vi "WriteConsumerState.vi"(8 "error in (no error)":errorcluster, 10 "Consumer State":string, 11 "Queue in":refnum<queue>) -> (0 "error out":errorcluster, 3 "Queue out":refnum<queue>)   [LabVIEW 2019]
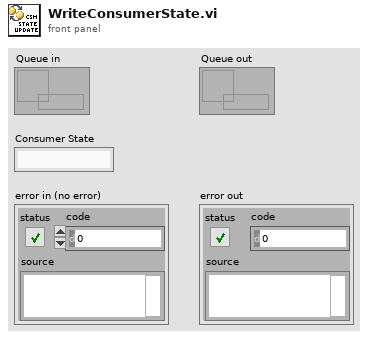
[diagram p1: front panel]
types:
  T1 = cluster{"Consumer State":string, "RxData":string, "error constant":errorcluster}
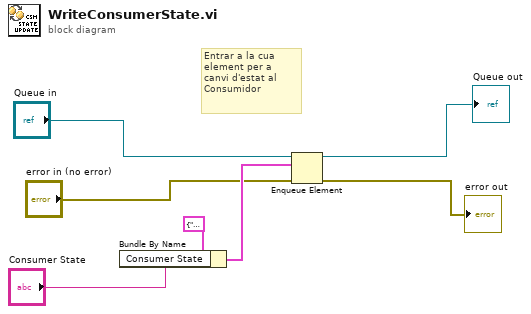
[diagram p0: block diagram]
diagram:
  # "Entrar a la cua element per a canvi d'estat al Consumidor"
  n1 = Bundle By Name(cluster=T1 {"Consumer State"="Consumer State", "RxData"="Received Data", "error constant"={"status"=FALSE, "code"=0, "source"=""}} ("Cluster 2"), "Consumer State"="Consumer State") -> (w6:T1)
  n2 = Enqueue Element(queue="Queue in", element=w6, error in (no error)="error in (no error)") -> (queue out=→"Queue out":refnum<queue>, error out=→"error out":errorcluster)  [unwired: 1 in, 1 out]
